vi "Run Runnable.vi"(8 "error in (no error)":errorcluster, 10 "Runnable":refnum<class "Runnable.lvclass">, 11 "Single Thread Test Runner In":refnum<class "Single Thread Test Runner.lvclass">) -> (0 "error out":errorcluster, 3 "Single Thread Test Runner Out":refnum<class "Single Thread Test Runner.lvclass">)   [LabVIEW 2020, in "Single Thread Test Runner.lvclass"]
uses:
  Single Thread Test Runner.lvclass
  Core/Runnable/Runnable.lvclass
  Execute.vi
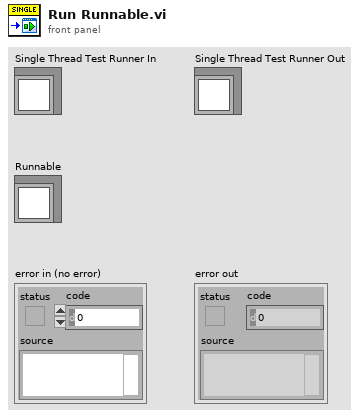
[diagram p1: front panel]
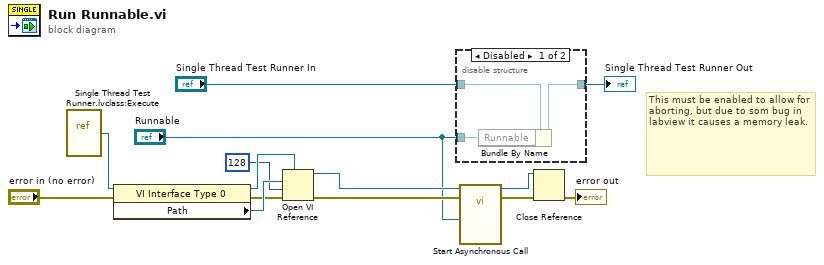
[diagram p0: block diagram]
diagram:
  # "This must be enabled to allow for aborting, but due to som bug in labview it causes a memory leak."
  n1 = vi-ref "Single Thread Test Runner.lvclass:Execute.vi"() -> (w14:refnum<vi>)
  n2 = property class="VI Interface Type 0"(reference=w14, error in="error in (no error)") -> (reference out=w12:refnum<vi>, error out=w11:errorcluster, "Path"=w13:path)
  n3 = Open VI Reference(type specifier VI Refnum (for type only)=w12, vi path=w13, options=128, error in (no error)=w11) -> (vi reference=w9:refnum<vi>, error out=w8:errorcluster)  [unwired: 2 in]
  n4 = disable-structure shown="Disabled" {
    disable-tunnel: "Single Thread Test Runner In" -> [w17 w18]
    disable-tunnel: [w16 w18] -> w2
    disable-tunnel: "Runnable" -> [w15 _]
    frame Disabled {
      n5 = Bundle By Name(cluster=w17, "Runnable"=w15) -> (w16:refnum<class "Single Thread Test Runner.lvclass">)
    }
    frame Enabled {
    }
  }
  "Single Thread Test Runner Out" <- w2
  n6 = call-by-ref "Start Asynchronous Call"(reference=w9, error in=w8, "Test Runner V2 in"="Runnable") -> (reference out=w7:refnum<vi>, error out=w6:errorcluster)  [unwired: 11 in]
  n7 = Close Reference(reference=w7, error in (no error)=w6) -> (error out=→"error out":errorcluster)
